vi "Do.vi"(8 "error in":errorcluster, 10 "Actor in":refnum<class "Actor.lvclass">, 11 "Check File Size MSG":refnum<class "Check File Size MSG.lvclass">) -> (0 "error out":errorcluster, 2 "Actor out":refnum<class "Actor.lvclass">)   [LabVIEW 2017, in "File Library.lvlib" / "Check File Size MSG.lvclass"]
doc: "(<B>Filename</B>: Actor Framework.lvlib:Message.lvclass:Do.vi)\n\nDefines what a message does when it is received by an actor. Generally, a message instructs an actor to invoke one of its methods. By default, this method does nothing. A child class must override it to define behavior. Create a child class by using the Actor Framework Message Maker dialog box."
uses:
  Check File Size MSG.lvclass
  <vilib>/ActorFramework/Actor/Actor.lvclass
  File Actor.lvclass
  C:/Program Files (x86)/National Instruments/LabVIEW 2017/vi.lib/ActorFramework/Actor/Actor.lvclass
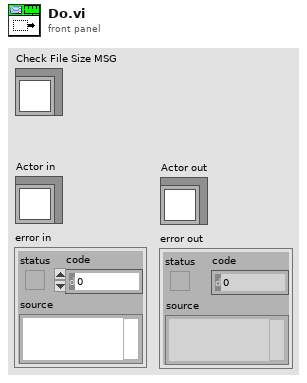
[diagram p1: front panel]
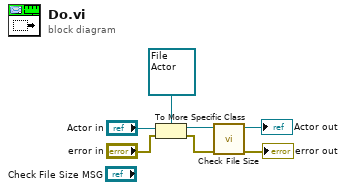
[diagram p0: block diagram]
diagram:
  n1 = To More Specific Class(target class=refnum<class "File Actor.lvclass"> refnum ("File Library.lvlib:File Actor"), reference="Actor in", error in="error in") -> (specific class reference=w4:refnum<class "File Actor.lvclass">, error out=w3:errorcluster)
  n2 = call "Check File Size.vi"("error in"=w3, "File Actor in"=w4) -> ("error out"=→"error out":errorcluster, "File Actor out"=→"Actor out":refnum<class "File Actor.lvclass">)  [unwired: 8 in]
